vi "Get Disable.vi"(8 "error in (no error)":errorcluster, 11 "S4ACS_GUI in":refnum<class "S4GUI.lvclass">) -> (0 "error out":errorcluster, 3 "S4ACS_GUI out":refnum<class "S4GUI.lvclass">)   [LabVIEW 2018, in "S4GUI.lvclass"]
uses:
  S4GUI.lvclass
  S4GUI.lvclass/S4GUI.ctl
  Server/Server.lvclass/Server.ctl
  Acquisition/Acquisition.lvclass
  C:/Users/devstaff/sparc4/s4gui/Versao ZeroMQ REQ-REP/SPARC4_GUI -20241016_20241016/Server/Server.lvclass
  Instrument/Instrument.lvclass
  Server/Server.lvclass
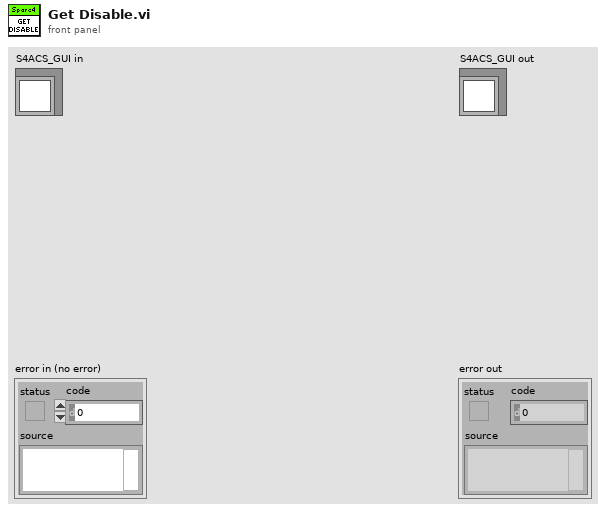
[diagram p1: front panel]
types:
  T1 = enum8{"Enabled", "Disabled", "Disabled and Grayed Out"}
  T2 = cluster{"Cluster Mode Sync":cluster{"#Index Cycles":enum8{"Enabled", "Disabled", "Disabled and Grayed Out"}, "#Cycles":enum8{"Enabled", "Disabled", "Disabled and Grayed Out"}, "SSM":enum8{"Enabled", "Disabled", "Disabled and Grayed Out"}, "Set SM":enum8{"Enabled", "Disabled", "Disabled and Grayed Out"}, "Star SM":enum8{"Enabled", "Disabled", "Disabled and Grayed Out"}, "Pause SM":enum8{"Enabled", "Disabled", "Disabled and Grayed Out"}, "Stop SM":enum8{"Enabled", "Disabled", "Disabled and Grayed Out"}, "Abort SM":enum8{"Enabled", "Disabled", "Disabled and Grayed Out"}, "Start SM Text":string}, "Cluster Polarimetry":cluster{"Lambda Selector":enum8{"Enabled", "Disabled", "Disabled and Grayed Out"}, "Calibrator Selector":enum8{"Enabled", "Disabled", "Disabled and Grayed Out"}, "Set Waveplate":enum8{"Enabled", "Disabled", "Disabled and Grayed Out"}, "Select Positions":enum8{"Enabled", "Disabled", "Disabled and Grayed Out"}, "P0":enum8{"Enabled", "Disabled", "Disabled and Grayed Out"}, "P1":enum8{"Enabled", "Disabled", "Disabled and Grayed Out"}, "P2":enum8{"Enabled", "Disabled", "Disabled and Grayed Out"}, "P3":enum8{"Enabled", "Disabled", "Disabled and Grayed Out"}, "P4":enum8{"Enabled", "Disabled", "Disabled and Grayed Out"}, "P5":enum8{"Enabled", "Disabled", "Disabled and Grayed Out"}, "P6":enum8{"Enabled", "Disabled", "Disabled and Grayed Out"}, "P7":enum8{"Enabled", "Disabled", "Disabled and Grayed Out"}, "P8":enum8{"Enabled", "Disabled", "Disabled and Grayed Out"}, "P9":enum8{"Enabled", "Disabled", "Disabled and Grayed Out"}, "P10":enum8{"Enabled", "Disabled", "Disabled and Grayed Out"}, "P11":enum8{"Enabled", "Disabled", "Disabled and Grayed Out"}, "P12":enum8{"Enabled", "Disabled", "Disabled and Grayed Out"}, "P13":enum8{"Enabled", "Disabled", "Disabled and Grayed Out"}, "P14":enum8{"Enabled", "Disabled", "Disabled and Grayed Out"}, "P15":enum8{"Enabled", "Disabled", "Disabled and Grayed Out"}}, "Cluster Mode CH1":cluster{"#cycles ch1":enum8{"Enabled", "Disabled", "Disabled and Grayed Out"}, "Start ch1":enum8{"Enabled", "Disabled", "Disabled and Grayed Out"}, "Pause ch1":enum8{"Enabled", "Disabled", "Disabled and Grayed Out"}, "Stop ch1":enum8{"Enabled", "Disabled", "Disabled and Grayed Out"}, "Abort ch1":enum8{"Enabled", "Disabled", "Disabled and Grayed Out"}, "Exptime ch1":enum8{"Enabled", "Disabled", "Disabled and Grayed Out"}, "Exp ch1":enum8{"Enabled", "Disabled", "Disabled and Grayed Out"}, "Start ch1 Text":string, "Set Cooler":enum8{"Enabled", "Disabled", "Disabled and Grayed Out"}, "Set Temp":enum8{"Enabled", "Disabled", "Disabled and Grayed Out"}}, "Cluster Mode CH2":cluster{"#cycles ch2":enum8{"Enabled", "Disabled", "Disabled and Grayed Out"}, "Start ch2":enum8{"Enabled", "Disabled", "Disabled and Grayed Out"}, "Pause ch2":enum8{"Enabled", "Disabled", "Disabled and Grayed Out"}, "Stop ch2":enum8{"Enabled", "Disabled", "Disabled and Grayed Out"}, "Abort ch2":enum8{"Enabled", "Disabled", "Disabled and Grayed Out"}, "Exptime ch2":enum8{"Enabled", "Disabled", "Disabled and Grayed Out"}, "Exp ch2":enum8{"Enabled", "Disabled", "Disabled and Grayed Out"}, "Start ch2 Text":string, "Set Cooler":enum8{"Enabled", "Disabled", "Disabled and Grayed Out"}, "Set Temp":enum8{"Enabled", "Disabled", "Disabled and Grayed Out"}}, "Cluster Mode CH3":cluster{"#cycles ch3":enum8{"Enabled", "Disabled", "Disabled and Grayed Out"}, "Start ch3":enum8{"Enabled", "Disabled", "Disabled and Grayed Out"}, "Pause ch3":enum8{"Enabled", "Disabled", "Disabled and Grayed Out"}, "Stop ch3":enum8{"Enabled", "Disabled", "Disabled and Grayed Out"}, "Abort ch3":enum8{"Enabled", "Disabled", "Disabled and Grayed Out"}, "Exptime ch3":enum8{"Enabled", "Disabled", "Disabled and Grayed Out"}, "Exp ch3":enum8{"Enabled", "Disabled", "Disabled and Grayed Out"}, "Start ch3 Text":string, "Set Cooler":enum8{"Enabled", "Disabled", "Disabled and Grayed Out"}, "Set Temp":enum8{"Enabled", "Disabled", "Disabled and Grayed Out"}}, "Cluster Mode CH4":cluster{"#cycles ch4":enum8{"Enabled", "Disabled", "Disabled and Grayed Out"}, "Start ch4":enum8{"Enabled", "Disabled", "Disabled and Grayed Out"}, "Pause ch4":enum8{"Enabled", "Disabled", "Disabled and Grayed Out"}, "Stop ch4":enum8{"Enabled", "Disabled", "Disabled and Grayed Out"}, "Abort ch4":enum8{"Enabled", "Disabled", "Disabled and Grayed Out"}, "Exptime ch4":enum8{"Enabled", "Disabled", "Disabled and Grayed Out"}, "Exp ch4":enum8{"Enabled", "Disabled", "Disabled and Grayed Out"}, "Start ch4 Text":string, "Set Cooler":enum8{"Enabled", "Disabled", "Disabled and Grayed Out"}, "Set Temp":enum8{"Enabled", "Disabled", "Disabled and Grayed Out"}}, "Cluster ExpMode":cluster{"tab4":enum8{"Enabled", "Disabled", "Disabled and Grayed Out"}}, "Cluster AdmCCDsetup":cluster{"param":enum8{"Enabled", "Disabled", "Disabled and Grayed Out"}}}
  T3 = enum32{"OBJECT", "DFLAT", "SFLAT", "DARK", "ZERO", "FOCUS"}
  T4 = cluster{"#Index Cycles":enum8{"Enabled", "Disabled", "Disabled and Grayed Out"}, "#Cycles":enum8{"Enabled", "Disabled", "Disabled and Grayed Out"}, "SSM":enum8{"Enabled", "Disabled", "Disabled and Grayed Out"}, "Set SM":enum8{"Enabled", "Disabled", "Disabled and Grayed Out"}, "Star SM":enum8{"Enabled", "Disabled", "Disabled and Grayed Out"}, "Pause SM":enum8{"Enabled", "Disabled", "Disabled and Grayed Out"}, "Stop SM":enum8{"Enabled", "Disabled", "Disabled and Grayed Out"}, "Abort SM":enum8{"Enabled", "Disabled", "Disabled and Grayed Out"}, "Start SM Text":string}
  T5 = cluster{"#cycles ch1":enum8{"Enabled", "Disabled", "Disabled and Grayed Out"}, "Start ch1":enum8{"Enabled", "Disabled", "Disabled and Grayed Out"}, "Pause ch1":enum8{"Enabled", "Disabled", "Disabled and Grayed Out"}, "Stop ch1":enum8{"Enabled", "Disabled", "Disabled and Grayed Out"}, "Abort ch1":enum8{"Enabled", "Disabled", "Disabled and Grayed Out"}, "Exptime ch1":enum8{"Enabled", "Disabled", "Disabled and Grayed Out"}, "Exp ch1":enum8{"Enabled", "Disabled", "Disabled and Grayed Out"}, "Start ch1 Text":string, "Set Cooler":enum8{"Enabled", "Disabled", "Disabled and Grayed Out"}, "Set Temp":enum8{"Enabled", "Disabled", "Disabled and Grayed Out"}}
  T6 = cluster{"#cycles ch2":enum8{"Enabled", "Disabled", "Disabled and Grayed Out"}, "Start ch2":enum8{"Enabled", "Disabled", "Disabled and Grayed Out"}, "Pause ch2":enum8{"Enabled", "Disabled", "Disabled and Grayed Out"}, "Stop ch2":enum8{"Enabled", "Disabled", "Disabled and Grayed Out"}, "Abort ch2":enum8{"Enabled", "Disabled", "Disabled and Grayed Out"}, "Exptime ch2":enum8{"Enabled", "Disabled", "Disabled and Grayed Out"}, "Exp ch2":enum8{"Enabled", "Disabled", "Disabled and Grayed Out"}, "Start ch2 Text":string, "Set Cooler":enum8{"Enabled", "Disabled", "Disabled and Grayed Out"}, "Set Temp":enum8{"Enabled", "Disabled", "Disabled and Grayed Out"}}
  T7 = cluster{"#cycles ch3":enum8{"Enabled", "Disabled", "Disabled and Grayed Out"}, "Start ch3":enum8{"Enabled", "Disabled", "Disabled and Grayed Out"}, "Pause ch3":enum8{"Enabled", "Disabled", "Disabled and Grayed Out"}, "Stop ch3":enum8{"Enabled", "Disabled", "Disabled and Grayed Out"}, "Abort ch3":enum8{"Enabled", "Disabled", "Disabled and Grayed Out"}, "Exptime ch3":enum8{"Enabled", "Disabled", "Disabled and Grayed Out"}, "Exp ch3":enum8{"Enabled", "Disabled", "Disabled and Grayed Out"}, "Start ch3 Text":string, "Set Cooler":enum8{"Enabled", "Disabled", "Disabled and Grayed Out"}, "Set Temp":enum8{"Enabled", "Disabled", "Disabled and Grayed Out"}}
  T8 = cluster{"#cycles ch4":enum8{"Enabled", "Disabled", "Disabled and Grayed Out"}, "Start ch4":enum8{"Enabled", "Disabled", "Disabled and Grayed Out"}, "Pause ch4":enum8{"Enabled", "Disabled", "Disabled and Grayed Out"}, "Stop ch4":enum8{"Enabled", "Disabled", "Disabled and Grayed Out"}, "Abort ch4":enum8{"Enabled", "Disabled", "Disabled and Grayed Out"}, "Exptime ch4":enum8{"Enabled", "Disabled", "Disabled and Grayed Out"}, "Exp ch4":enum8{"Enabled", "Disabled", "Disabled and Grayed Out"}, "Start ch4 Text":string, "Set Cooler":enum8{"Enabled", "Disabled", "Disabled and Grayed Out"}, "Set Temp":enum8{"Enabled", "Disabled", "Disabled and Grayed Out"}}
  T9 = cluster{"Lambda Selector":enum8{"Enabled", "Disabled", "Disabled and Grayed Out"}, "Calibrator Selector":enum8{"Enabled", "Disabled", "Disabled and Grayed Out"}, "Set Waveplate":enum8{"Enabled", "Disabled", "Disabled and Grayed Out"}, "Select Positions":enum8{"Enabled", "Disabled", "Disabled and Grayed Out"}, "P0":enum8{"Enabled", "Disabled", "Disabled and Grayed Out"}, "P1":enum8{"Enabled", "Disabled", "Disabled and Grayed Out"}, "P2":enum8{"Enabled", "Disabled", "Disabled and Grayed Out"}, "P3":enum8{"Enabled", "Disabled", "Disabled and Grayed Out"}, "P4":enum8{"Enabled", "Disabled", "Disabled and Grayed Out"}, "P5":enum8{"Enabled", "Disabled", "Disabled and Grayed Out"}, "P6":enum8{"Enabled", "Disabled", "Disabled and Grayed Out"}, "P7":enum8{"Enabled", "Disabled", "Disabled and Grayed Out"}, "P8":enum8{"Enabled", "Disabled", "Disabled and Grayed Out"}, "P9":enum8{"Enabled", "Disabled", "Disabled and Grayed Out"}, "P10":enum8{"Enabled", "Disabled", "Disabled and Grayed Out"}, "P11":enum8{"Enabled", "Disabled", "Disabled and Grayed Out"}, "P12":enum8{"Enabled", "Disabled", "Disabled and Grayed Out"}, "P13":enum8{"Enabled", "Disabled", "Disabled and Grayed Out"}, "P14":enum8{"Enabled", "Disabled", "Disabled and Grayed Out"}, "P15":enum8{"Enabled", "Disabled", "Disabled and Grayed Out"}}
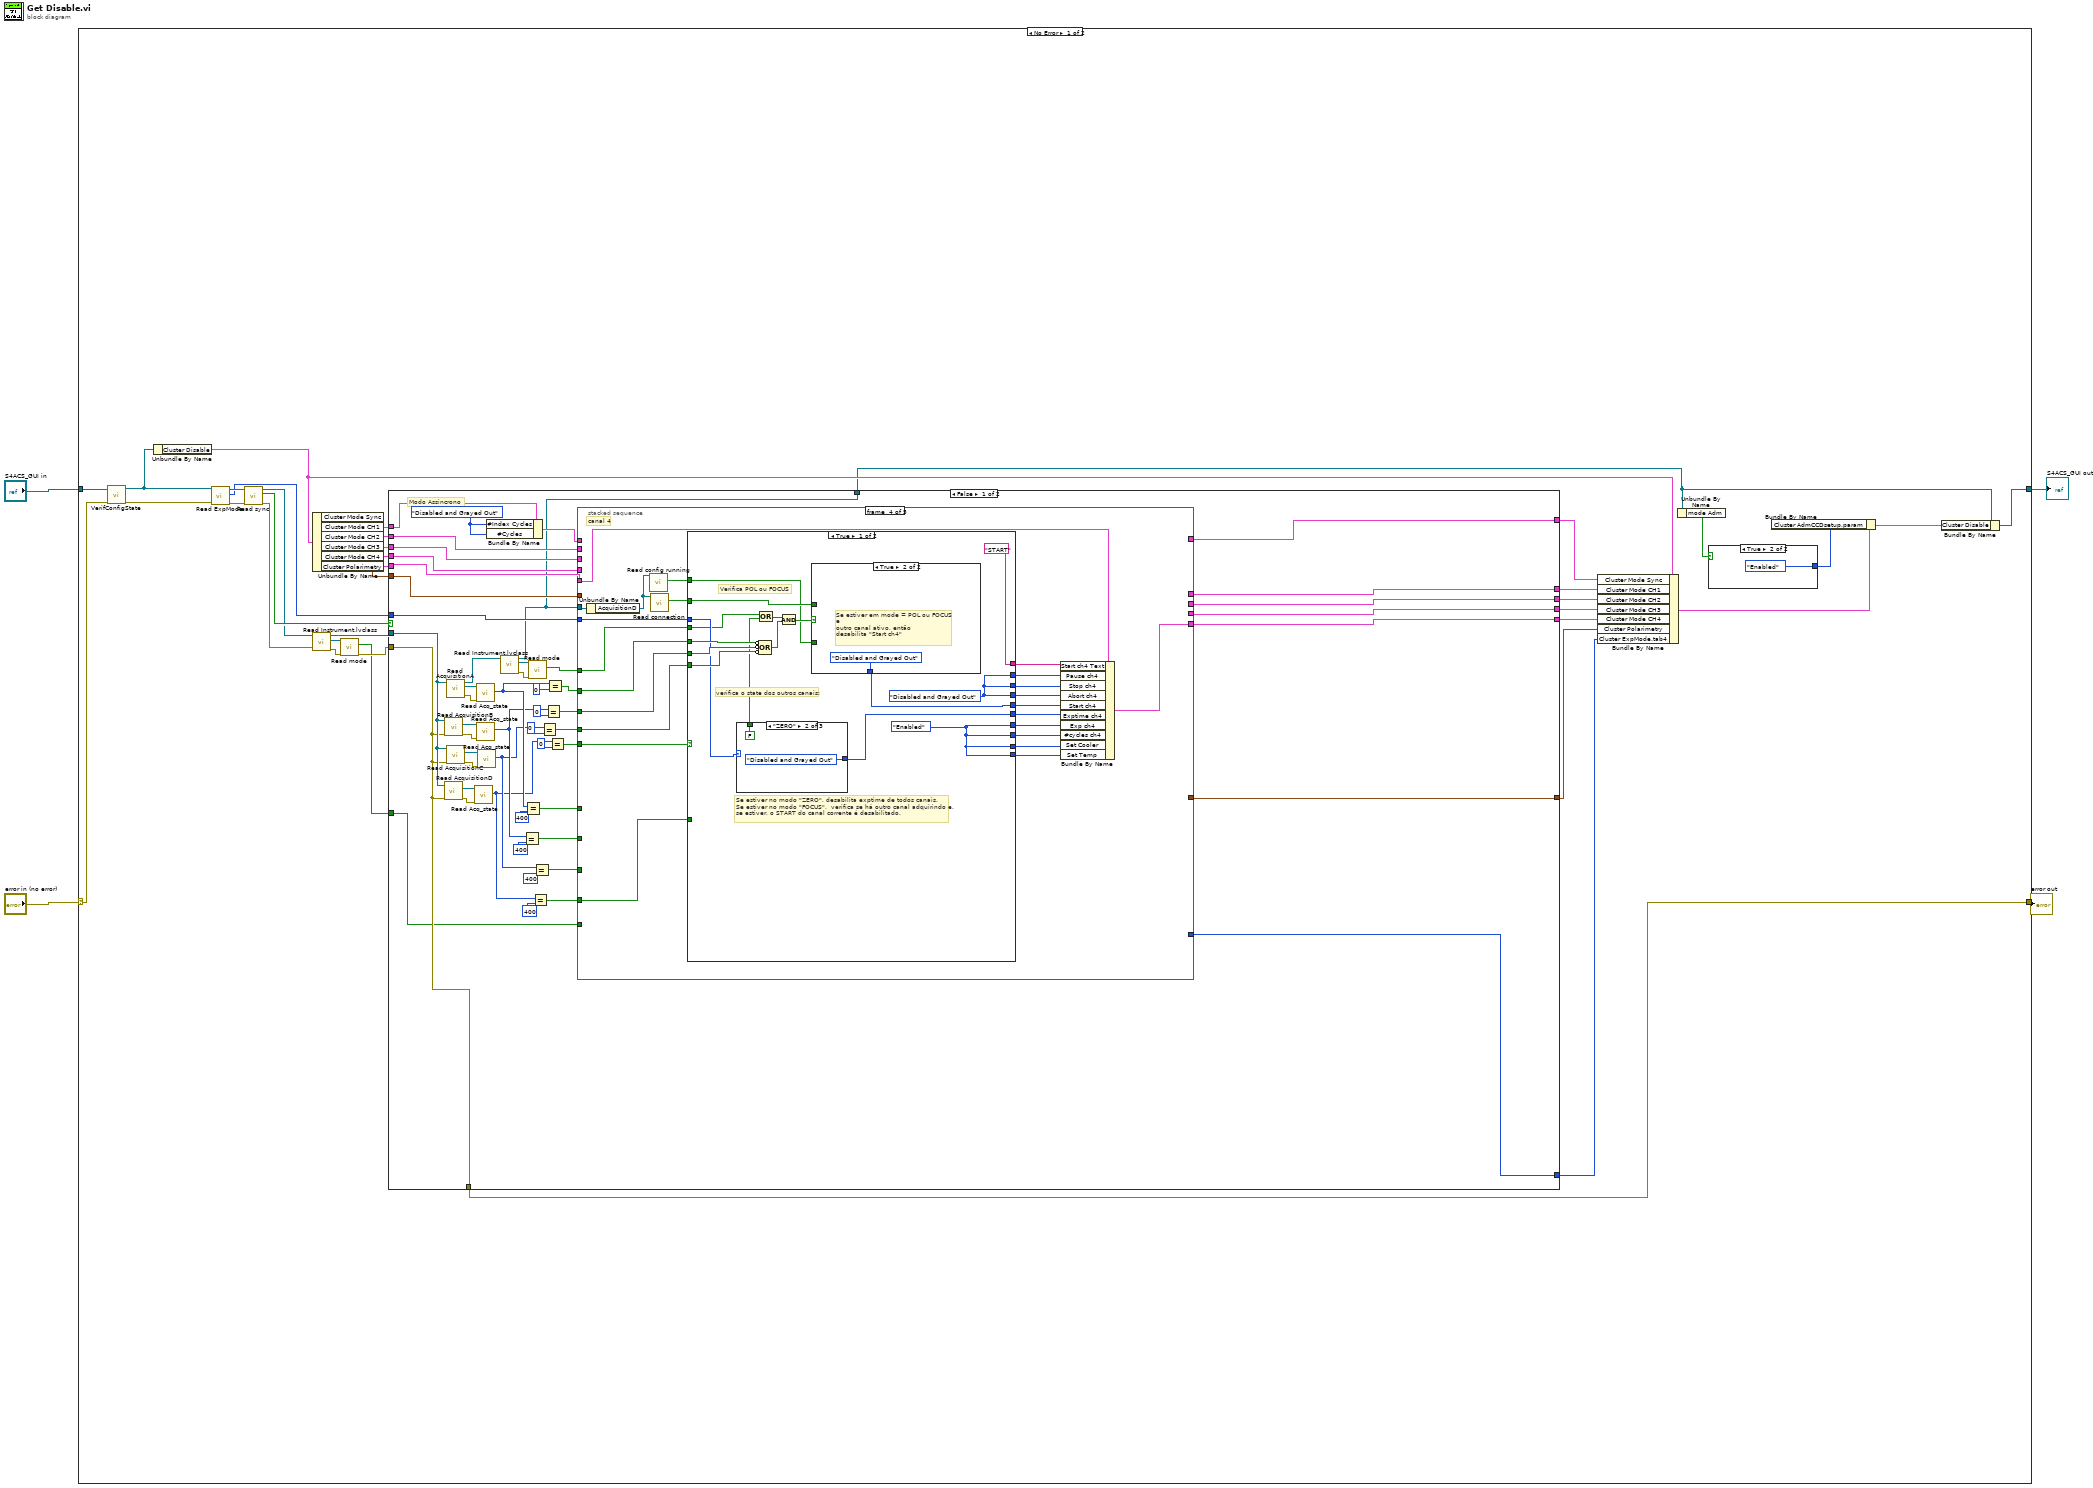
[diagram p0: block diagram]
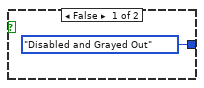
[diagram p2: hidden frame]
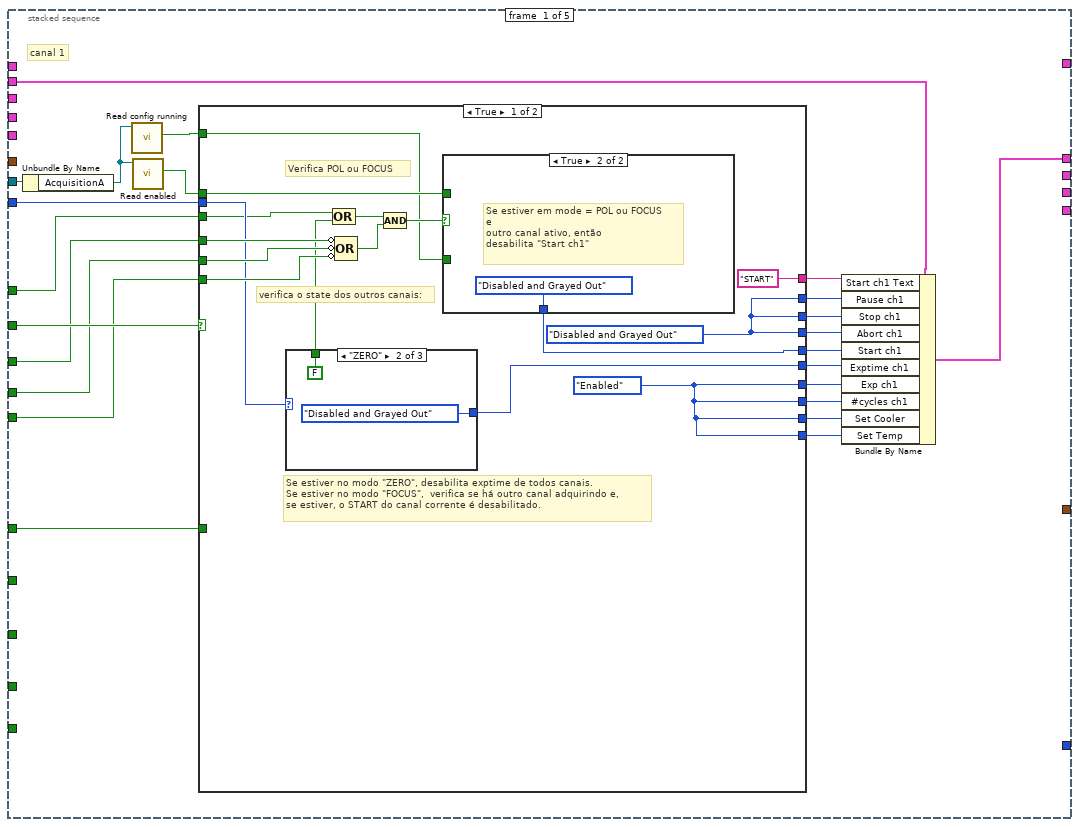
[diagram p3: hidden frame]
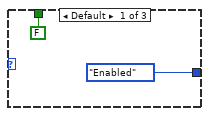
[diagram p4: hidden frame]
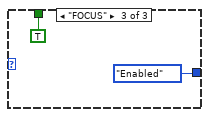
[diagram p5: hidden frame]
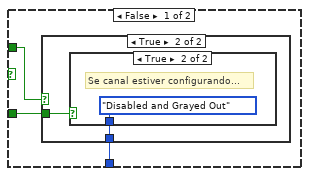
[diagram p6: hidden frame]
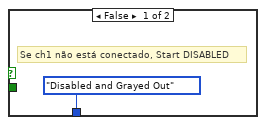
[diagram p7: hidden frame]
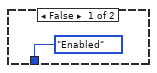
[diagram p8: hidden frame]
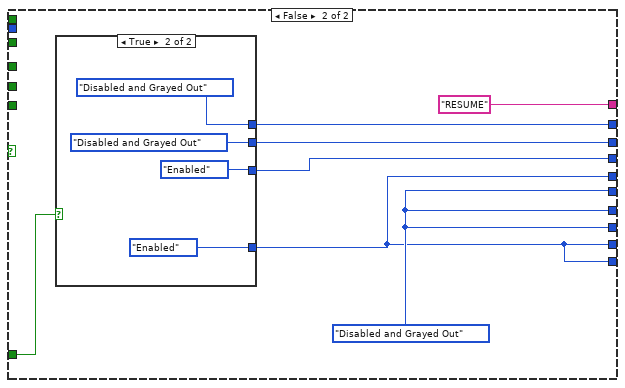
[diagram p9: hidden frame]
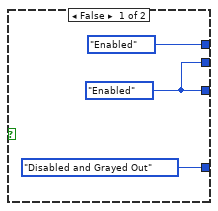
[diagram p10: hidden frame]
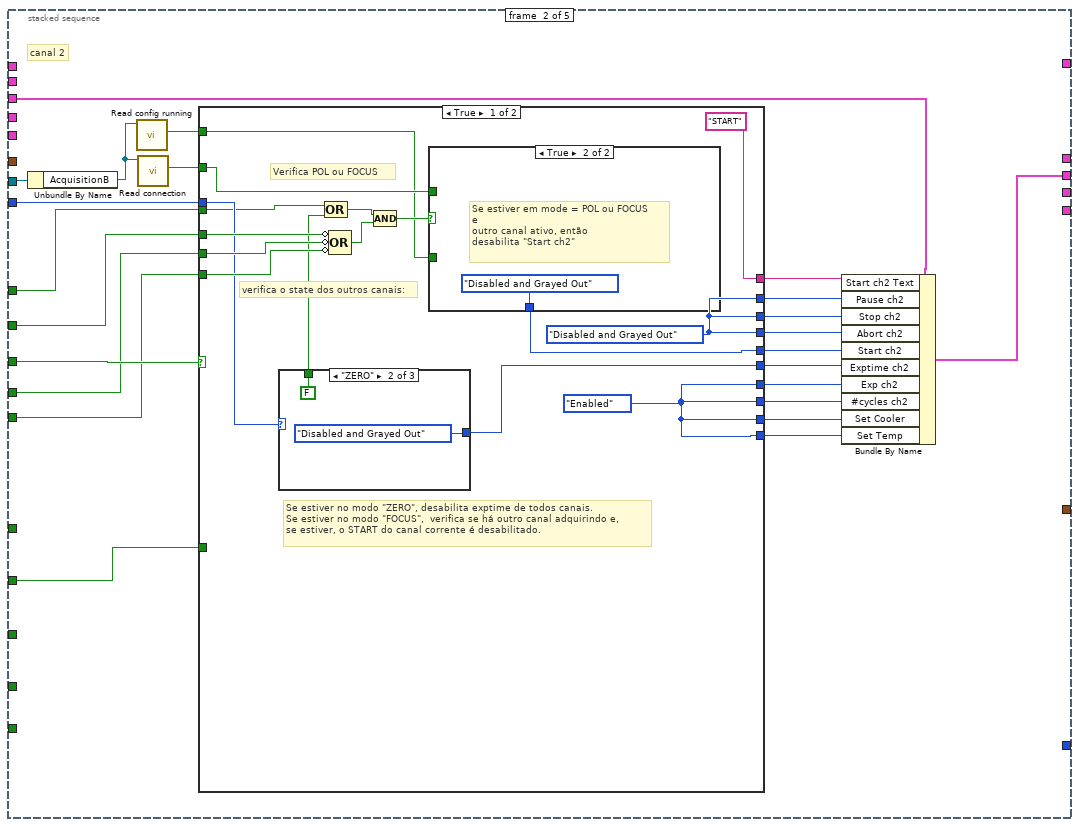
[diagram p11: hidden frame]
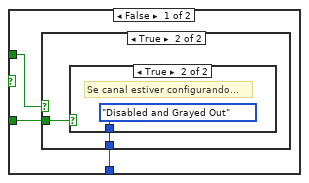
[diagram p12: hidden frame]
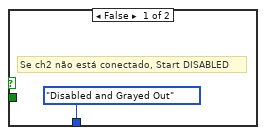
[diagram p13: hidden frame]
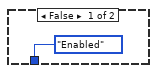
[diagram p14: hidden frame]
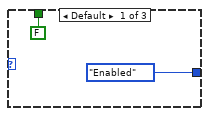
[diagram p15: hidden frame]
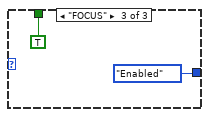
[diagram p16: hidden frame]
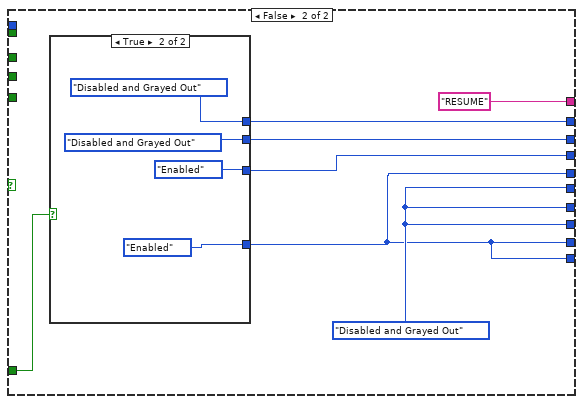
[diagram p17: hidden frame]
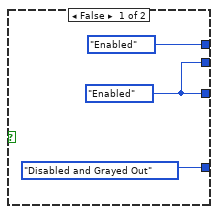
[diagram p18: hidden frame]
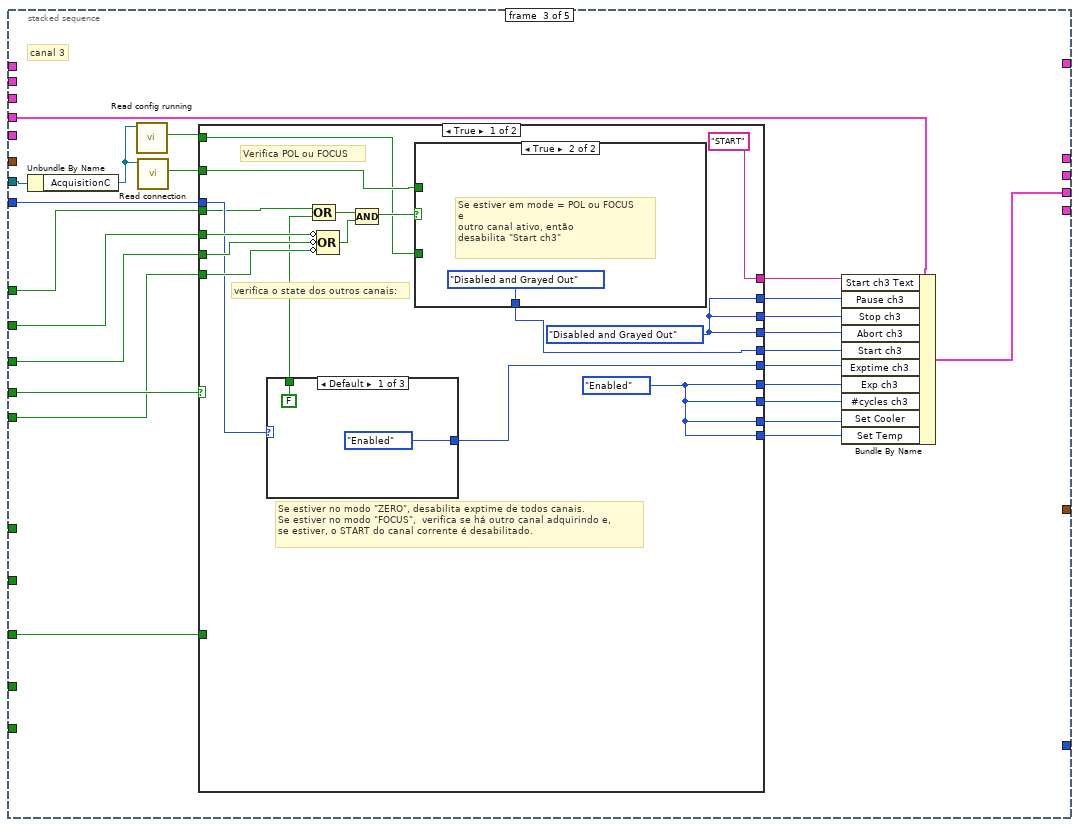
[diagram p19: hidden frame]
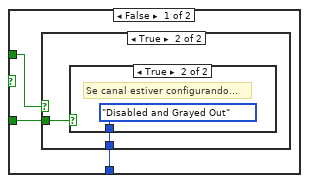
[diagram p20: hidden frame]
diagram:
  n1 = case shown="No Error" "error in (no error)" {
    selector: "error in (no error)" -> [w21 w513]
    tunnel: [w33 w513] -> w3
    tunnel: [w5 w512] -> w1
    tunnel: "S4ACS_GUI in" -> [w22 w512]
    frame No Error {
      n2 = call-dynamic "VerifConfigState.vi"("error in (no error)"=w21, "S4GUI in"=w22) -> ("error out"=w9:errorcluster, "S4GUI out"=w8:refnum<class "S4GUI.lvclass">)  [unwired: 8 in]
      n3 = Unbundle By Name(w8) -> ("Cluster Disable"=w7:T2)
      n4 = call-dynamic "Read ExpMode.vi"("error in (no error)"=w9, "S4GUI in"=w8) -> ("error out"=w24:errorcluster, "ExpMode"=w23:T3, "S4GUI out"=w25:refnum<class "S4GUI.lvclass">)  [unwired: 7 in]
      n5 = call-dynamic "Read sync.vi"("error in (no error)"=w24, "S4ACS_GUI in"=w25) -> ("error out"=w14:errorcluster, "sync"=w40:bool, "S4ACS_GUI out"=w16:refnum<class "S4GUI.lvclass">)  [unwired: 7 in]
      n6 = Unbundle By Name(w7) -> ("Cluster Mode Sync"=w39:T4, "Cluster Mode CH1"=w38:T5, "Cluster Mode CH2"=w37:T6, "Cluster Mode CH3"=w31:T7, "Cluster Mode CH4"=w30:T8, "Cluster Polarimetry"=w32:T9)
      n7 = call "Read Instrument.lvclass.vi"("error in (no error)"=w14, "S4ACS_GUI in"=w16) -> ("error out"=w13:errorcluster, "Instrument.lvclass"=w17:refnum<class "Instrument.lvclass">, "S4ACS_GUI out"=w15:refnum<class "S4GUI.lvclass">)  [unwired: 7 in]
      n8 = call-dynamic "Read mode.vi"("error in (no error)"=w13, "Instrument in"=w17) -> ("error out"=w12:errorcluster, "mode"=w11:bool)  [unwired: 7 in, 1 out]
      n9 = case shown="False" w40 {
        tunnel: w15 -> [w63 w445]
        tunnel: w12 -> [w62 w444]
        tunnel: w39 -> [w76 w443]
        tunnel: w38 -> [w74 w435]
        tunnel: w37 -> [w72 w432]
        tunnel: [w73 w441] -> w36
        tunnel: [w51 w433] -> w35
        tunnel: w32 -> [w71 w440]
        tunnel: [w70 w431] -> w29
        tunnel: [w50 w434] -> w34
        tunnel: [w62 w430] -> w33
        tunnel: [w46 w413] -> w6
        tunnel: w31 -> [w69 w426]
        tunnel: w30 -> [w68 w422]
        tunnel: [w49 w425] -> w28
        tunnel: [w48 w421] -> w27
        tunnel: [w45 w420] -> w26
        tunnel: w23 -> [w47 w419]
        tunnel: w11 -> [w43 w408]
        frame False {
          w44 = T1."Disabled and Grayed Out" ("Disabled")
          # "Modo Assincrono"
          n10 = call-dynamic "Read AcquisitionD.vi"("error in (no error)"=w62, "S4ACS_GUI in"=w63) -> ("error out"=w64:errorcluster, "Acquisition.lvclass"=w65:refnum<class "Acquisition.lvclass">)  [unwired: 7 in, 1 out]
          n11 = call "Read AcquisitionB.vi"("error in (no error)"=w62, "S4ACS_GUI in"=w63) -> ("error out"=w91:errorcluster, "Acquisition.lvclass"=w92:refnum<class "Acquisition.lvclass">)  [unwired: 7 in, 1 out]
          n12 = call-dynamic "Read AcquisitionC.vi"("error in (no error)"=w62, "S4ACS_GUI in"=w63) -> ("error out"=w67:errorcluster, "Acquisition.lvclass"=w66:refnum<class "Acquisition.lvclass">)  [unwired: 7 in, 1 out]
          n13 = call-dynamic "Read AcquisitionA.vi"("S4ACS_GUI in"=w63) -> ("error out"=w93:errorcluster, "Acquisition.lvclass"=w94:refnum<class "Acquisition.lvclass">, "S4ACS_GUI out"=w77:refnum<class "S4GUI.lvclass">)  [unwired: 8 in]
          n14 = call-dynamic "Read Acq_state.vi"("error in (no error)"=w64, "Acquisition in"=w65) -> ("Acq_state"=w54:u32)  [unwired: 7 in, 2 out]
          n15 = call-dynamic "Read Acq_state.vi"("error in (no error)"=w93, "Acquisition in"=w94) -> ("Acq_state"=w84:u32)  [unwired: 7 in, 2 out]
          n16 = call-dynamic "Read Acq_state.vi"("error in (no error)"=w91, "Acquisition in"=w92) -> ("Acq_state"=w81:u32)  [unwired: 7 in, 2 out]
          n17 = call-dynamic "Read Acq_state.vi"("error in (no error)"=w67, "Acquisition in"=w66) -> ("Acq_state"=w55:u32)  [unwired: 7 in, 2 out]
          n18 = Bundle By Name(cluster=w76, "#Index Cycles"=w44, "#Cycles"=w44) -> (w75:T4)
          n19 = call "Read Instrument.lvclass.vi"("S4ACS_GUI in"=w77) -> ("error out"=w79:errorcluster, "Instrument.lvclass"=w80:refnum<class "Instrument.lvclass">, "S4ACS_GUI out"=w46:refnum<class "S4GUI.lvclass">)  [unwired: 8 in]
          n20 = Equal?(x=w81, y=u32 400) -> (x = y?=w85:bool)
          n21 = Equal?(x=w84, y=u32 400) -> (x = y?=w86:bool)
          n22 = call-dynamic "Read mode.vi"("error in (no error)"=w79, "Instrument in"=w80) -> ("mode"=w78:bool)  [unwired: 7 in, 2 out]
          n23 = Equal?(x=w54, y=u32 400) -> (x = y?=w52:bool)
          n24 = Equal?(x=w55, y=u32 400) -> (x = y?=w53:bool)
          n25 = Equal?(x=w55, y=u32 0) -> (x = y?=w59:bool)
          n26 = Equal?(x=w81, y=u32 0) -> (x = y?=w83:bool)
          n27 = Equal?(x=w84, y=u32 0) -> (x = y?=w89:bool)
          n28 = Equal?(x=w54, y=u32 0) -> (x = y?=w60:bool)
          n29 = stacked-sequence {
            tunnel: w89 -> [w117 w174 w244 w312 w401]
            tunnel: w86 -> [w116 _ _ _ w399]
            tunnel: w85 -> [_ w172 _ _ w398]
            tunnel: w83 -> [w114 w173 w241 w308 w400]
            tunnel: w78 -> [w115 w185 w253 w321 _]
            tunnel: w75 -> [_ _ _ _ w393]
            tunnel: w74 -> [w113 _ _ _ _]
            tunnel: [_ _ _ _ w392] -> w73
            tunnel: [w104 _ _ _ _] -> w51
            tunnel: w72 -> [_ w176 _ _ _]
            tunnel: w71 -> [_ _ _ _ w395]
            tunnel: [_ _ _ _ w394] -> w70
            tunnel: [_ w175 _ _ _] -> w50
            tunnel: w69 -> [_ _ w243 _ _]
            tunnel: w68 -> [_ _ _ w311 _]
            tunnel: [_ _ w242 _ _] -> w49
            tunnel: [_ _ _ w310 _] -> w48
            tunnel: w59 -> [w103 w171 w240 w307 w389]
            tunnel: w60 -> [w102 w170 w239 w309 w388]
            tunnel: w53 -> [_ _ w238 _ w387]
            tunnel: w52 -> [_ _ _ w306 w386]
            tunnel: w47 -> [w101 w169 w237 w305 _]
            tunnel: w46 -> [w98 w165 w233 w302 w382]
            tunnel: [_ _ _ _ w385] -> w45
            tunnel: w43 -> [_ _ _ _ w383]
            frame #0 {
              # "canal 1"
              n30 = Unbundle By Name(w98) -> ("AcquisitionA"=w96:refnum<class "Acquisition.lvclass">)
              n31 = call-dynamic "Read config running.vi"("Server in"=w96) -> ("config running"=w95:bool)  [unwired: 8 in, 2 out]
              n32 = call-dynamic "Read enabled.vi"("Server in"=w96) -> ("enabled"=w97:bool)  [unwired: 8 in, 2 out]
              n33 = case shown="True" w117 {
                tunnel: w116 -> [_ w155]
                tunnel: w115 -> [w120 _]
                tunnel: w114 -> [w129 _]
                tunnel: ["START" ("Caption.Text") "RESUME" ("Caption.Text")] -> w112
                tunnel: [w131 w153] -> w111
                tunnel: [w131 w149] -> w110
                tunnel: [w131 w150] -> w109
                tunnel: [w130 w151] -> w108
                tunnel: [w124 w152] -> w107
                tunnel: [w123 w152] -> w106
                tunnel: [w123 w152] -> w105
                tunnel: w103 -> [w128 _]
                tunnel: w102 -> [w127 _]
                tunnel: w101 -> [w125 _]
                tunnel: [w123 w151] -> w100
                tunnel: [w123 w151] -> w99
                tunnel: w97 -> [w122 _]
                tunnel: w95 -> [w121 _]
                frame True {
                  w131 = T1."Disabled and Grayed Out" ("Disabled")
                  w123 = T1."Enabled" ("Disabled")
                  # "Verifica POL ou FOCUS"
                  # "Se estiver no modo \"ZERO\", desabilita exptime de todos canais.\nSe estiver no modo \"FOCUS\",  verifica se há outro canal adquirindo e,\nse estiver, o START do canal corrente é desabilitado."
                  # "verifica o state dos outros canais:"
                  n34 = case shown="\"ZERO\"" w125 {
                    tunnel: [T1."Enabled" ("Disabled") T1."Disabled and Grayed Out" ("Disabled") T1."Enabled" ("Disabled")] -> w124
                    tunnel: [FALSE FALSE TRUE] -> w118
                    frame Default {
                    }
                    frame "ZERO" {
                    }
                    frame "FOCUS" {
                    }
                  }
                  n35 = Compound Arithmetic op=OR(w120, w118) -> (w119:bool)
                  n36 = Compound Arithmetic op=OR(invert w129, invert w128, invert w127) -> (w126:bool)
                  n37 = Compound Arithmetic op=AND(w119, w126) -> (w133:bool)
                  n38 = case shown="True" w133 {
                    tunnel: [w142 T1."Disabled and Grayed Out" ("Disabled")] -> w130
                    tunnel: w122 -> [w141 _]
                    tunnel: w121 -> [w140 _]
                    frame False {
                      n39 = case shown="True" w141 {
                        tunnel: [T1."Disabled and Grayed Out" ("Disabled") w145] -> w142
                        tunnel: w140 -> [_ w144]
                        frame False {
                          # "Se ch1 não está conectado, Start DISABLED"
                        }
                        frame True {
                          n40 = case shown="True" w144 {
                            tunnel: [T1."Enabled" ("Disabled") T1."Disabled and Grayed Out" ("Disabled")] -> w145
                            frame False {
                            }
                            frame True {
                              # "Se canal estiver configurando..."
                            }
                          }
                        }
                      }
                    }
                    frame True {
                      # "Se estiver em mode = POL ou FOCUS\ne\noutro canal ativo, então\ndesabilita \"Start ch1\""
                    }
                  }
                }
                frame False {
                  w152 = T1."Disabled and Grayed Out" ("Disabled")
                  n41 = case shown="True" w155 {
                    tunnel: [T1."Enabled" ("Disabled") T1."Disabled and Grayed Out" ("Disabled")] -> w153
                    tunnel: [T1."Disabled and Grayed Out" ("Disabled") T1."Enabled" ("Disabled")] -> w151
                    tunnel: [w156 T1."Enabled" ("Disabled")] -> w150
                    tunnel: [w156 T1."Disabled and Grayed Out" ("Disabled")] -> w149
                    frame False {
                      w156 = T1."Enabled" ("Disabled")
                    }
                    frame True {
                    }
                  }
                }
              }
              n42 = Bundle By Name(cluster=w113, "Start ch1 Text"=w112, "Pause ch1"=w111, "Stop ch1"=w110, "Abort ch1"=w109, "Start ch1"=w108, "Exptime ch1"=w107, "Exp ch1"=w106, "#cycles ch1"=w105, "Set Cooler"=w100, "Set Temp"=w99) -> (w104:T5)
            }
            frame #1 {
              # "canal 2"
              n43 = Unbundle By Name(w165) -> ("AcquisitionB"=w166:refnum<class "Acquisition.lvclass">)
              n44 = call-dynamic "Read config running.vi"("Server in"=w166) -> ("config running"=w163:bool)  [unwired: 8 in, 2 out]
              n45 = call "Read connection.vi"("Server in"=w166) -> ("connection"=w164:bool)  [unwired: 8 in, 2 out]
              n46 = case shown="True" w173 {
                tunnel: w172 -> [_ w221]
                tunnel: w185 -> [w186 _]
                tunnel: w174 -> [w198 _]
                tunnel: ["START" ("Caption.Text") "RESUME" ("Caption.Text")] -> w184
                tunnel: [w200 w219] -> w183
                tunnel: [w200 w218] -> w182
                tunnel: [w200 w217] -> w181
                tunnel: [w189 w220] -> w180
                tunnel: [w194 w222] -> w179
                tunnel: [w193 w222] -> w178
                tunnel: [w193 w222] -> w177
                tunnel: w171 -> [w197 _]
                tunnel: w170 -> [w196 _]
                tunnel: w169 -> [w195 _]
                tunnel: [w193 w220] -> w168
                tunnel: [w193 w220] -> w167
                tunnel: w164 -> [w191 _]
                tunnel: w163 -> [w190 _]
                frame True {
                  w200 = T1."Disabled and Grayed Out" ("Disabled")
                  w193 = T1."Enabled" ("Disabled")
                  # "Verifica POL ou FOCUS"
                  # "Se estiver no modo \"ZERO\", desabilita exptime de todos canais.\nSe estiver no modo \"FOCUS\",  verifica se há outro canal adquirindo e,\nse estiver, o START do canal corrente é desabilitado."
                  # "verifica o state dos outros canais:"
                  n47 = case shown="\"ZERO\"" w195 {
                    tunnel: [T1."Enabled" ("Disabled") T1."Disabled and Grayed Out" ("Disabled") T1."Enabled" ("Disabled")] -> w194
                    tunnel: [FALSE FALSE TRUE] -> w187
                    frame Default {
                    }
                    frame "ZERO" {
                    }
                    frame "FOCUS" {
                    }
                  }
                  n48 = Compound Arithmetic op=OR(w186, w187) -> (w188:bool)
                  n49 = Compound Arithmetic op=OR(invert w198, invert w197, invert w196) -> (w199:bool)
                  n50 = Compound Arithmetic op=AND(w188, w199) -> (w192:bool)
                  n51 = case shown="True" w192 {
                    tunnel: [w204 T1."Disabled and Grayed Out" ("Disabled")] -> w189
                    tunnel: w191 -> [w203 _]
                    tunnel: w190 -> [w202 _]
                    frame False {
                      n52 = case shown="True" w203 {
                        tunnel: [T1."Disabled and Grayed Out" ("Disabled") w207] -> w204
                        tunnel: w202 -> [_ w206]
                        frame False {
                          # "Se ch2 não está conectado, Start DISABLED"
                        }
                        frame True {
                          n53 = case shown="True" w206 {
                            tunnel: [T1."Enabled" ("Disabled") T1."Disabled and Grayed Out" ("Disabled")] -> w207
                            frame False {
                            }
                            frame True {
                              # "Se canal estiver configurando..."
                            }
                          }
                        }
                      }
                    }
                    frame True {
                      # "Se estiver em mode = POL ou FOCUS\ne\noutro canal ativo, então\ndesabilita \"Start ch2\""
                    }
                  }
                }
                frame False {
                  w222 = T1."Disabled and Grayed Out" ("Disabled")
                  n54 = case shown="True" w221 {
                    tunnel: [T1."Enabled" ("Disabled") T1."Disabled and Grayed Out" ("Disabled")] -> w219
                    tunnel: [T1."Disabled and Grayed Out" ("Disabled") T1."Enabled" ("Disabled")] -> w220
                    tunnel: [w224 T1."Enabled" ("Disabled")] -> w217
                    tunnel: [w224 T1."Disabled and Grayed Out" ("Disabled")] -> w218
                    frame False {
                      w224 = T1."Enabled" ("Disabled")
                    }
                    frame True {
                    }
                  }
                }
              }
              n55 = Bundle By Name(cluster=w176, "Start ch2 Text"=w184, "Pause ch2"=w183, "Stop ch2"=w182, "Abort ch2"=w181, "Start ch2"=w180, "Exptime ch2"=w179, "Exp ch2"=w178, "#cycles ch2"=w177, "Set Cooler"=w168, "Set Temp"=w167) -> (w175:T6)
            }
            frame #2 {
              # "canal 3"
              n56 = Unbundle By Name(w233) -> ("AcquisitionC"=w234:refnum<class "Acquisition.lvclass">)
              n57 = call-dynamic "Read config running.vi"("Server in"=w234) -> ("config running"=w231:bool)  [unwired: 8 in, 2 out]
              n58 = call "Read connection.vi"("Server in"=w234) -> ("connection"=w232:bool)  [unwired: 8 in, 2 out]
              n59 = case shown="True" w240 {
                tunnel: w238 -> [_ w289]
                tunnel: w253 -> [w255 _]
                tunnel: w244 -> [w266 _]
                tunnel: ["START" ("Caption.Text") "RESUME" ("Caption.Text")] -> w252
                tunnel: [w268 w288] -> w251
                tunnel: [w268 w286] -> w250
                tunnel: [w268 w285] -> w249
                tunnel: [w260 w287] -> w248
                tunnel: [w262 w290] -> w247
                tunnel: [w261 w290] -> w246
                tunnel: [w261 w290] -> w245
                tunnel: w241 -> [w265 _]
                tunnel: w239 -> [w264 _]
                tunnel: w237 -> [w263 _]
                tunnel: [w261 w287] -> w236
                tunnel: [w261 w287] -> w235
                tunnel: w232 -> [w258 _]
                tunnel: w231 -> [w257 _]
                frame True {
                  w268 = T1."Disabled and Grayed Out" ("Disabled")
                  w261 = T1."Enabled" ("Disabled")
                  # "Verifica POL ou FOCUS"
                  # "Se estiver no modo \"ZERO\", desabilita exptime de todos canais.\nSe estiver no modo \"FOCUS\",  verifica se há outro canal adquirindo e,\nse estiver, o START do canal corrente é desabilitado."
                  # "verifica o state dos outros canais:"
                  n60 = case shown="Default" w263 {
                    tunnel: [T1."Enabled" ("Disabled") T1."Disabled and Grayed Out" ("Disabled") T1."Enabled" ("Disabled")] -> w262
                    tunnel: [FALSE FALSE TRUE] -> w254
                    frame Default {
                    }
                    frame "ZERO" {
                    }
                    frame "FOCUS" {
                    }
                  }
                  n61 = Compound Arithmetic op=OR(w255, w254) -> (w256:bool)
                  n62 = Compound Arithmetic op=OR(invert w266, invert w265, invert w264) -> (w267:bool)
                  n63 = Compound Arithmetic op=AND(w256, w267) -> (w259:bool)
                  n64 = case shown="True" w259 {
                    tunnel: [w272 T1."Disabled and Grayed Out" ("Disabled")] -> w260
                    tunnel: w258 -> [w271 _]
                    tunnel: w257 -> [w270 _]
                    frame False {
                      n65 = case shown="True" w271 {
                        tunnel: [T1."Disabled and Grayed Out" ("Disabled") w275] -> w272
                        tunnel: w270 -> [_ w274]
                        frame False {
                          # "Se ch3 não está conectado, Start DISABLED"
                        }
                        frame True {
                          n66 = case shown="True" w274 {
                            tunnel: [T1."Enabled" ("Disabled") T1."Disabled and Grayed Out" ("Disabled")] -> w275
                            frame False {
                            }
                            frame True {
                              # "Se canal estiver configurando..."
                            }
                          }
                        }
                      }
                    }
                    frame True {
                      # "Se estiver em mode = POL ou FOCUS\ne\noutro canal ativo, então\ndesabilita \"Start ch3\""
                    }
                  }
                }
                frame False {
                  w290 = T1."Disabled and Grayed Out" ("Disabled")
                  n67 = case shown="True" w289 {
                    tunnel: [T1."Enabled" ("Disabled") T1."Disabled and Grayed Out" ("Disabled")] -> w288
                    tunnel: [T1."Disabled and Grayed Out" ("Disabled") T1."Enabled" ("Disabled")] -> w287
                    tunnel: [w292 T1."Enabled" ("Disabled")] -> w285
                    tunnel: [w292 T1."Disabled and Grayed Out" ("Disabled")] -> w286
                    frame False {
                      w292 = T1."Enabled" ("Disabled")
                    }
                    frame True {
                    }
                  }
                }
              }
              n68 = Bundle By Name(cluster=w243, "Start ch3 Text"=w252, "Pause ch3"=w251, "Stop ch3"=w250, "Abort ch3"=w249, "Start ch3"=w248, "Exptime ch3"=w247, "Exp ch3"=w246, "#cycles ch3"=w245, "Set Cooler"=w236, "Set Temp"=w235) -> (w242:T7)
            }
            frame #3 {
              # "canal 4"
              n69 = Unbundle By Name(w302) -> ("AcquisitionD"=w301:refnum<class "Acquisition.lvclass">)
              n70 = call-dynamic "Read config running.vi"("Server in"=w301) -> ("config running"=w300:bool)  [unwired: 8 in, 2 out]
              n71 = call "Read connection.vi"("Server in"=w301) -> ("connection"=w299:bool)  [unwired: 8 in, 2 out]
              n72 = case shown="True" w309 {
                tunnel: w306 -> [_ w355]
                tunnel: w321 -> [w322 _]
                tunnel: w312 -> [w334 _]
                tunnel: ["START" ("Caption.Text") "RESUME" ("Caption.Text")] -> w320
                tunnel: [w336 w357] -> w319
                tunnel: [w336 w354] -> w318
                tunnel: [w336 w353] -> w317
                tunnel: [w328 w356] -> w316
                tunnel: [w330 w358] -> w315
                tunnel: [w329 w358] -> w314
                tunnel: [w329 w358] -> w313
                tunnel: w308 -> [w333 _]
                tunnel: w307 -> [w332 _]
                tunnel: w305 -> [w331 _]
                tunnel: [w329 w356] -> w304
                tunnel: [w329 w356] -> w303
                tunnel: w300 -> [w325 _]
                tunnel: w299 -> [w326 _]
                frame True {
                  w336 = T1."Disabled and Grayed Out" ("Disabled")
                  w329 = T1."Enabled" ("Disabled")
                  # "Verifica POL ou FOCUS"
                  # "Se estiver no modo \"ZERO\", desabilita exptime de todos canais.\nSe estiver no modo \"FOCUS\",  verifica se há outro canal adquirindo e,\nse estiver, o START do canal corrente é desabilitado."
                  # "verifica o state dos outros canais:"
                  n73 = case shown="\"ZERO\"" w331 {
                    tunnel: [T1."Enabled" ("Disabled") T1."Disabled and Grayed Out" ("Disabled") T1."Enabled" ("Disabled")] -> w330
                    tunnel: [FALSE FALSE TRUE] -> w323
                    frame Default {
                    }
                    frame "ZERO" {
                    }
                    frame "FOCUS" {
                    }
                  }
                  n74 = Compound Arithmetic op=OR(invert w334, invert w333, invert w332) -> (w335:bool)
                  n75 = Compound Arithmetic op=OR(w322, w323) -> (w324:bool)
                  n76 = Compound Arithmetic op=AND(w324, w335) -> (w327:bool)
                  n77 = case shown="True" w327 {
                    tunnel: [w340 T1."Disabled and Grayed Out" ("Disabled")] -> w328
                    tunnel: w326 -> [w339 _]
                    tunnel: w325 -> [w338 _]
                    frame False {
                      n78 = case shown="False" w339 {
                        tunnel: [T1."Disabled and Grayed Out" ("Disabled") w343] -> w340
                        tunnel: w338 -> [_ w342]
                        frame False {
                          # "Se ch4 não está conectado, Start DISABLED"
                        }
                        frame True {
                          n79 = case shown="False" w342 {
                            tunnel: [T1."Enabled" ("Disabled") T1."Disabled and Grayed Out" ("Disabled")] -> w343
                            frame False {
                            }
                            frame True {
                              # "Se canal estiver configurando..."
                            }
                          }
                        }
                      }
                    }
                    frame True {
                      # "Se estiver em mode = POL ou FOCUS\ne\noutro canal ativo, então\ndesabilita \"Start ch4\""
                    }
                  }
                }
                frame False {
                  w358 = T1."Disabled and Grayed Out" ("Disabled")
                  n80 = case shown="True" w355 {
                    tunnel: [T1."Enabled" ("Disabled") T1."Disabled and Grayed Out" ("Disabled")] -> w357
                    tunnel: [T1."Disabled and Grayed Out" ("Disabled") T1."Enabled" ("Disabled")] -> w356
                    tunnel: [w360 T1."Enabled" ("Disabled")] -> w353
                    tunnel: [w360 T1."Disabled and Grayed Out" ("Disabled")] -> w354
                    frame False {
                      w360 = T1."Enabled" ("Disabled")
                    }
                    frame True {
                    }
                  }
                }
              }
              n81 = Bundle By Name(cluster=w311, "Start ch4 Text"=w320, "Pause ch4"=w319, "Stop ch4"=w318, "Abort ch4"=w317, "Start ch4"=w316, "Exptime ch4"=w315, "Exp ch4"=w314, "#cycles ch4"=w313, "Set Cooler"=w304, "Set Temp"=w303) -> (w310:T8)
            }
            frame #4 {
              w390 = T1."Disabled and Grayed Out" ("Disabled")
              # "Se algum canal está sendo \nconfigurado,  desabilita \nbotão SET."
              # "Se algum canal está adquirindo, \ndesabilita botão SET."
              # "comum a todos os canais"
              n82 = Compound Arithmetic op=AND(w399, w398, w387, w386) -> (w396:bool)
              n83 = Compound Arithmetic op=AND(w401, w400, w389, w388) -> (w371:bool)
              n84 = Or(x=w371, y=w396) -> (x .or. y?=w397:bool)
              n85 = case shown="True" w397 {
                tunnel: [w402 T1."Enabled" ("Disabled")] -> w385
                tunnel: [w402 w404] -> w384
                tunnel: w383 -> [_ w403]
                frame False {
                  w402 = T1."Disabled and Grayed Out" ("Disabled")
                }
                frame True {
                  n86 = case shown="False" w403 {
                    tunnel: [T1."Disabled and Grayed Out" ("Disabled") T1."Enabled" ("Disabled")] -> w404
                    frame False {
                      # "Photometric"
                    }
                    frame True {
                      # "Polarimetric"
                    }
                  }
                }
              }
              n87 = Unbundle By Name(w382) -> ("AcquisitionA"=w377:refnum<class "Acquisition.lvclass">)
              n88 = Unbundle By Name(w382) -> ("AcquisitionB"=w376:refnum<class "Acquisition.lvclass">)
              n89 = Unbundle By Name(w382) -> ("AcquisitionC"=w375:refnum<class "Acquisition.lvclass">)
              n90 = Unbundle By Name(w382) -> ("AcquisitionD"=w374:refnum<class "Acquisition.lvclass">)
              n91 = call-dynamic "Read config running.vi"("Server in"=w377) -> ("config running"=w381:bool)  [unwired: 8 in, 2 out]
              n92 = call-dynamic "Read config running.vi"("Server in"=w376) -> ("config running"=w380:bool)  [unwired: 8 in, 2 out]
              n93 = call-dynamic "Read config running.vi"("Server in"=w375) -> ("config running"=w379:bool)  [unwired: 8 in, 2 out]
              n94 = call-dynamic "Read config running.vi"("Server in"=w374) -> ("config running"=w378:bool)  [unwired: 8 in, 2 out]
              n95 = Select(t=T1."Enabled" ("Disabled"), s=w371, f=T1."Disabled and Grayed Out" ("Disabled")) -> (s? t:f=w368:T1)
              n96 = Compound Arithmetic op=OR(w381, w380, w379, w378) -> (w373:bool)
              n97 = Select(t=T1."Disabled and Grayed Out" ("Disabled"), s=w373, f=w368) -> (s? t:f=w367:T1)
              n98 = Bundle By Name(cluster=w393, "SSM"=w385, "Start SM Text"="START", "Star SM"=w390, "Pause SM"=w390, "Stop SM"=w390, "Abort SM"=w390, "Set SM"=w367) -> (w392:T4)
              n99 = Bundle By Name(cluster=w395, "P0"=w384, "P1"=w384, "P2"=w384, "P3"=w384, "P4"=w384, "P5"=w384, "P6"=w384, "P7"=w384, "P8"=w384, "P9"=w384, "P10"=w384, "P11"=w384, "P12"=w384, "P13"=w384, "P14"=w384, "P15"=w384, "Lambda Selector"=w385, "Calibrator Selector"=w385, "Set Waveplate"=w385, "Select Positions"=w384) -> (w394:T9)
            }
          }
        }
        frame True {
          w424 = T1."Disabled and Grayed Out" ("Disabled")
          # "Modo Síncrono"
          n100 = call-dynamic "Read Obs_state.vi"("error in (no error)"=w444, "S4ACS_GUI in"=w445) -> ("error out"=w430:errorcluster, "Obs_state"=w446:u32, "S4ACS_GUI out"=w413:refnum<class "S4GUI.lvclass">)  [unwired: 7 in]
          n101 = Equal?(x=w446, y=u32 0) -> (x = y?=w447:bool)
          n102 = case shown="True" w447 {
            tunnel: w446 -> [_ w496]
            tunnel: ["START" ("Caption.Text") "RESUME" ("Caption.Text")] -> w442
            tunnel: [w455 w498] -> w409
            tunnel: [w456 w498] -> w412
            tunnel: [w456 w498] -> w439
            tunnel: [w462 w497] -> w411
            tunnel: [w462 T1."Enabled" ("Disabled")] -> w438
            tunnel: [w462 w501] -> w437
            tunnel: [w453 w495] -> w436
            tunnel: [w458 w499] -> w417
            tunnel: [T1."Enabled" ("Disabled") T1."Disabled and Grayed Out" ("Disabled")] -> w420
            tunnel: w419 -> [w460 _]
            tunnel: [w459 w499] -> w418
            tunnel: [w458 w495] -> w416
            tunnel: [w458 w495] -> w415
            tunnel: [w456 w498] -> w414
            tunnel: w413 -> [w451 _]
            tunnel: w408 -> [w454 _]
            frame True {
              w458 = T1."Enabled" ("Disabled")
              w462 = T1."Disabled and Grayed Out" ("Disabled")
              # "Se estiver no modo \"ZERO\", desabilita exptime de todos canais."
              n103 = disable-structure shown="Enabled" {
                disable-tunnel: w451 -> [w473 w478]
                disable-tunnel: [w464 w483] -> w457
                frame Disabled {
                  n104 = Unbundle By Name(w473) -> ("AcquisitionA"=w472:refnum<class "Acquisition.lvclass">, "AcquisitionB"=w471:refnum<class "Acquisition.lvclass">, "AcquisitionC"=w470:refnum<class "Acquisition.lvclass">, "AcquisitionD"=w469:refnum<class "Acquisition.lvclass">)
                  n105 = call "Read connection.vi"("Server in"=w470) -> ("connection"=w466:bool)  [unwired: 8 in, 2 out]
                  n106 = call "Read connection.vi"("Server in"=w471) -> ("connection"=w467:bool)  [unwired: 8 in, 2 out]
                  n107 = call "Read connection.vi"("Server in"=w469) -> ("connection"=w465:bool)  [unwired: 8 in, 2 out]
                  n108 = call "Read connection.vi"("Server in"=w472) -> ("connection"=w468:bool)  [unwired: 8 in, 2 out]
                  n109 = Compound Arithmetic op=OR(w468, w467, w466, w465) -> (w464:bool)
                }
                frame Enabled {
                  n110 = Unbundle By Name(w478) -> ("AcquisitionA"=w477:refnum<class "Acquisition.lvclass">)
                  n111 = Unbundle By Name(w478) -> ("AcquisitionB"=w476:refnum<class "Acquisition.lvclass">)
                  n112 = Unbundle By Name(w478) -> ("AcquisitionC"=w475:refnum<class "Acquisition.lvclass">)
                  n113 = Unbundle By Name(w478) -> ("AcquisitionD"=w474:refnum<class "Acquisition.lvclass">)
                  n114 = call-dynamic "Read config running.vi"("Server in"=w477) -> ("config running"=w482:bool)  [unwired: 8 in, 2 out]
                  n115 = call-dynamic "Read config running.vi"("Server in"=w476) -> ("config running"=w481:bool)  [unwired: 8 in, 2 out]
                  n116 = call-dynamic "Read config running.vi"("Server in"=w475) -> ("config running"=w480:bool)  [unwired: 8 in, 2 out]
                  n117 = call-dynamic "Read config running.vi"("Server in"=w474) -> ("config running"=w479:bool)  [unwired: 8 in, 2 out]
                  n118 = Compound Arithmetic op=OR(w482, w481, w480, w479) -> (w483:bool)
                }
              }
              n119 = Unbundle By Name(w451) -> ("Error Msg"=w450:string)
              n120 = case shown="\"ZERO\"" w460 {
                tunnel: [T1."Disabled and Grayed Out" ("Disabled") T1."Enabled" ("Disabled")] -> w459
                frame "ZERO" {
                }
                frame Default {
                }
              }
              n121 = String Length(string=w450) -> (length=w452:i32)
              n122 = Greater Than 0?(x=w452) -> (x > 0?=w449:bool)
              n123 = case shown="False" w457 {
                tunnel: [w486 w492] -> w456
                tunnel: [w489 w492] -> w455
                tunnel: w454 -> [w488 _]
                tunnel: [w485 w492] -> w453
                tunnel: w449 -> [w487 _]
                frame False {
                  w486 = T1."Enabled" ("Disabled")
                  n124 = case shown="True" w488 {
                    tunnel: [T1."Disabled and Grayed Out" ("Disabled") T1."Enabled" ("Disabled")] -> w489
                    frame False {
                      # "Photometric"
                    }
                    frame True {
                      # "Polarimetric"
                    }
                  }
                  n125 = Select(t=T1."Disabled and Grayed Out" ("Disabled"), s=w487, f=w486) -> (s? t:f=w485:T1)
                }
                frame True {
                  w492 = T1."Disabled and Grayed Out" ("Disabled")
                }
              }
            }
            frame False {
              w499 = T1."Disabled and Grayed Out" ("Disabled")
              w498 = T1."Disabled and Grayed Out" ("Disabled")
              # "paused?"
              n126 = Equal?(x=w496, y=u32 400) -> (x = y?=w505:bool)
              n127 = case shown="True" w505 {
                tunnel: w498 -> [w508 w511]
                tunnel: [w508 T1."Enabled" ("Disabled")] -> w495
                tunnel: [T1."Enabled" ("Disabled") w511] -> w501
                tunnel: [T1."Enabled" ("Disabled") T1."Disabled and Grayed Out" ("Disabled")] -> w497
                frame False {
                }
                frame True {
                }
              }
            }
          }
          n128 = Bundle By Name(cluster=w443, "Start SM Text"=w442, "Star SM"=w436, "#Index Cycles"=T1."Enabled" ("Disabled"), "#Cycles"=w412, "Set SM"=w412, "SSM"=w414, "Pause SM"=w437, "Stop SM"=w411, "Abort SM"=w438) -> (w441:T4)
          n129 = Bundle By Name(cluster=w440, "P0"=w409, "P1"=w409, "P2"=w409, "P3"=w409, "P4"=w409, "P5"=w409, "P6"=w409, "P7"=w409, "P8"=w409, "P9"=w409, "P10"=w409, "P11"=w409, "P12"=w409, "P13"=w409, "P14"=w409, "P15"=w409, "Lambda Selector"=w439, "Calibrator Selector"=w439, "Set Waveplate"=w439, "Select Positions"=w409) -> (w431:T9)
          n130 = Bundle By Name(cluster=w435, "Exptime ch1"=w418, "Exp ch1"=w417, "#cycles ch1"=w424, "Start ch1 Text"="Sync", "Start ch1"=w424, "Pause ch1"=w424, "Stop ch1"=w424, "Abort ch1"=w424, "Set Cooler"=w416, "Set Temp"=w415) -> (w434:T5)
          n131 = Bundle By Name(cluster=w432, "Exptime ch2"=w418, "Exp ch2"=w417, "#cycles ch2"=w424, "Start ch2 Text"="Sync", "Start ch2"=w424, "Pause ch2"=w424, "Stop ch2"=w424, "Abort ch2"=w424, "Set Cooler"=w416, "Set Temp"=w415) -> (w433:T6)
          n132 = Bundle By Name(cluster=w426, "Exptime ch3"=w418, "Exp ch3"=w417, "#cycles ch3"=w424, "Start ch3 Text"="Sync" ("Start ch2 Text"), "Start ch3"=w424, "Pause ch3"=w424, "Stop ch3"=w424, "Abort ch3"=w424, "Set Cooler"=w416, "Set Temp"=w415) -> (w425:T7)
          n133 = Bundle By Name(cluster=w422, "Exptime ch4"=w418, "Exp ch4"=w417, "#cycles ch4"=w424, "Start ch4 Text"="Sync" ("Start ch2 Text"), "Start ch4"=w424, "Pause ch4"=w424, "Stop ch4"=w424, "Abort ch4"=w424, "Set Cooler"=w416, "Set Temp"=w415) -> (w421:T8)
        }
      }
      n134 = Bundle By Name(cluster=w7, "Cluster Mode Sync"=w36, "Cluster Mode CH1"=w35, "Cluster Mode CH2"=w34, "Cluster Mode CH3"=w28, "Cluster Mode CH4"=w27, "Cluster Polarimetry"=w29, "Cluster ExpMode.tab4"=w26) -> (w20:T2)
      n135 = Unbundle By Name(w6) -> ("mode Adm"=w19:bool)
      n136 = case shown="True" w19 {
        tunnel: [T1."Disabled and Grayed Out" ("Cluster AdmCCDSetup.param") T1."Enabled" ("Cluster AdmCCDSetup.param")] -> w18
        frame False {
        }
        frame True {
        }
      }
      n137 = Bundle By Name(cluster=w20, "Cluster AdmCCDsetup.param"=w18) -> (w10:T2)
      n138 = Bundle By Name(cluster=w6, "Cluster Disable"=w10) -> (w5:refnum<class "S4GUI.lvclass">)
    }
    frame Error {
    }
  }
  "error out" <- w3
  "S4ACS_GUI out" <- w1
